vi "用零补全4位数组.vi"(1 "数组输入":u16[](array[numeric])) -> (0 "数组输出":i32[](array[numeric]))   [LabVIEW 2013]
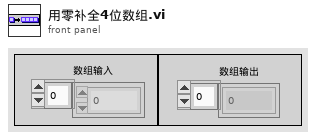
[diagram p1: front panel]
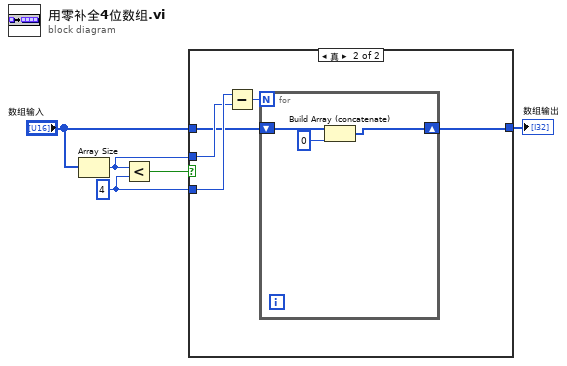
[diagram p0: block diagram]
diagram:
  w4 = 4 ("y")
  n1 = Array Size(array="数组输入") -> (size(s)=w3:i32)
  n2 = Less?(x=w3, y=w4) -> (x < y?=w5:bool)
  n3 = case shown="真" w5 {
    tunnel: w4 -> [_ w10]
    tunnel: w3 -> [_ w9]
    tunnel: [w6 w7] -> w1
    tunnel: "数组输入" -> [w6 w8]
    frame False {
    }
    frame True {
      n4 = Subtract(x=w10, y=w9) -> (x-y=w11:i32)
      n5 = for {
        N: w11 -> [_]
        shift-right: [w12] -> w7
        shift-left: w8 -> [w14]
        n6 = Build Array (concatenate)(w14, 0 ("y")) -> (w12:i32[])
      }
    }
  }
  "数组输出" <- w1
